vi "convert--duration to formatted string.vi"(1 "duration (seconds)":dbl format="%.3f") -> (0 "duration (formatted string)":string)   [LabVIEW 2020, in "core.lvlib"]
uses:
  core.lvlib
  core_data/chessboard_index.ctl
  core_data/core_data.lvlib
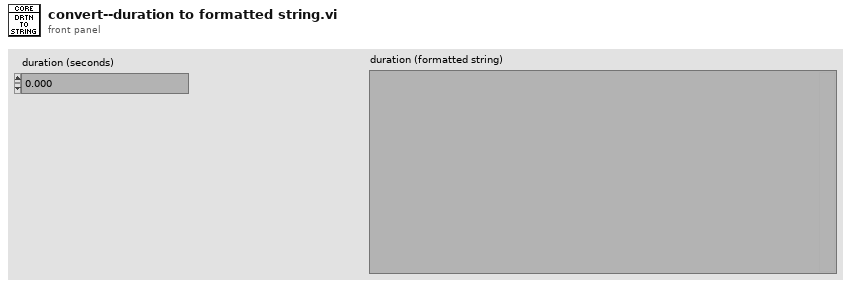
[diagram p1: front panel]
types:
  T1 = typedef "core.lvlib/core_data.lvlib/chessboard_index.ctl" = cluster{"row":u8, "column":u8}
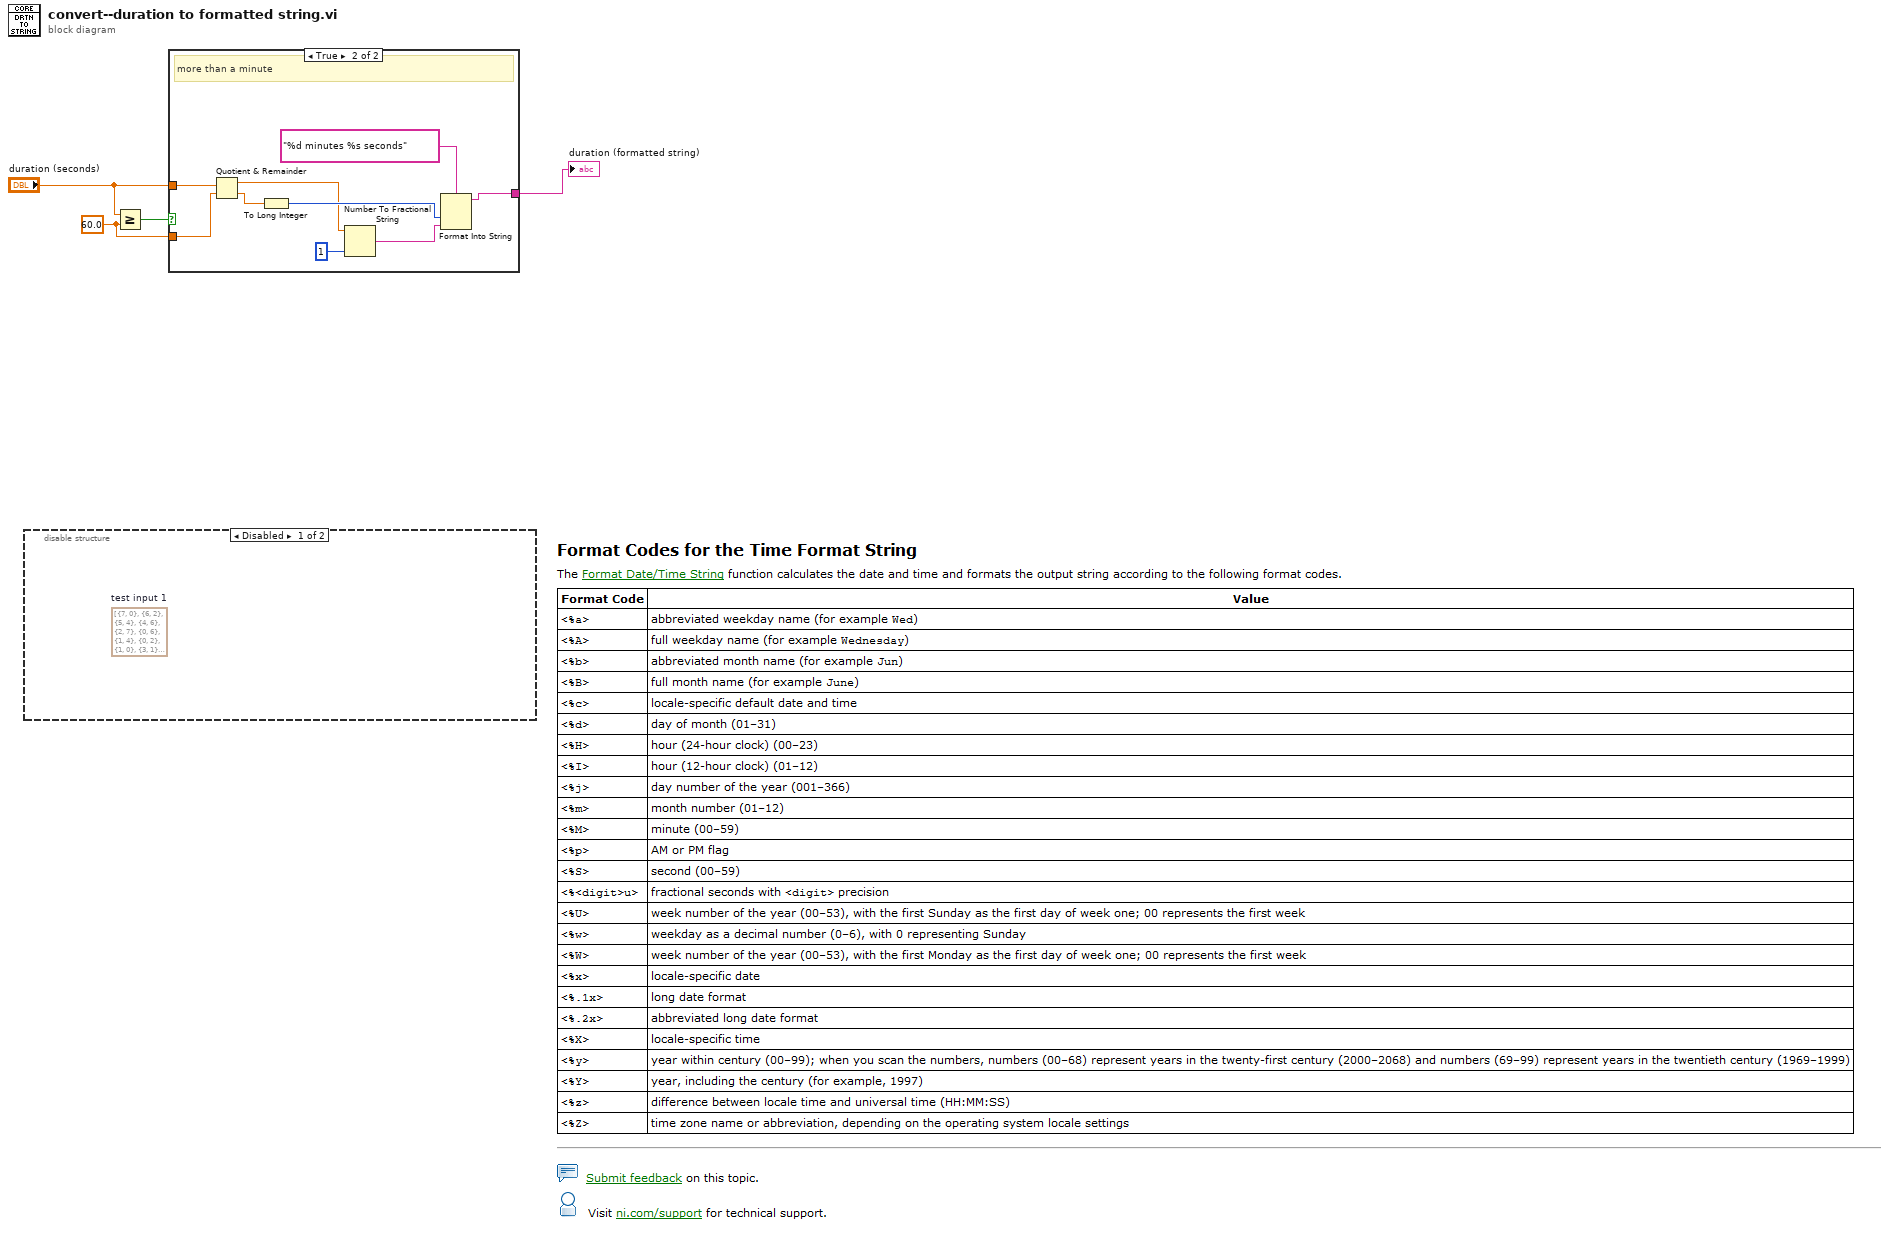
[diagram p0: block diagram]
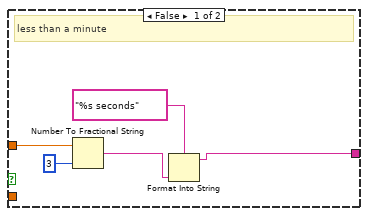
[diagram p2: hidden frame]
diagram:
  w1 = 60.0 ("y")
  n1 = disable-structure shown="Disabled" {
    frame Disabled {
      (unwired) T1[] [{"row"=7, "column"=0}, {"row"=6, "column"=2}, {"row"=5, "column"=4}, {"row"=4, "column"=6}, {"row"=2, "column"=7}, {"row"=0, "column"=6}, {"row"=1, "column"=4}, {"row"=0, "column"=2}, {"row"=1, "column"=0}, {"row"=3, "column"=1}, {"row"=2, "column"=3}, {"row"=1, "column"=5}, {"row"=0, "column"=7}, {"row"=2, "column"=6}, {"row"=0, "column"=5}, {"row"=1, "column"=3}, {"row"=0, "column"=1}, {"row"=2, "column"=0}, {"row"=1, "column"=2}, {"row"=0, "column"=4}, {"row"=2, "column"=5}, {"row"=1, "column"=7}, {"row"=3, "column"=6}, {"row"=2, "column"=4}, {"row"=1, "column"=6}, {"row"=3, "column"=5}, {"row"=4, "column"=3}, {"row"=2, "column"=2}, {"row"=0, "column"=3}, {"row"=1, "column"=1}, {"row"=3, "column"=0}, {"row"=5, "column"=1}, {"row"=3, "column"=2}]  # test input 1
    }
    frame Enabled {
    }
  }
  n2 = Greater Or Equal?(x="duration (seconds)", y=w1) -> (x >= y?=w2:bool)
  n3 = case shown="True" w2 {
    tunnel: "duration (seconds)" -> [w9 w18]
    tunnel: [w5 w10] -> w3
    tunnel: w1 -> [_ w17]
    frame False {
      # "less than a minute"
      n4 = Number To Fractional String(number=w9, precision (6)=i16 3) -> (F-format string=w6:string)  [unwired: 2 in]
      n5 = Format Into String(format string="%s seconds", w6) -> (resulting string=w5:string)  [unwired: 2 in, 1 out]
    }
    frame True {
      # "more than a minute"
      n6 = Quotient & Remainder(x=w18, y=w17) -> (x-y*floor(x/y)=w11:dbl, floor(x/y)=w14:dbl)
      n7 = To Long Integer(number=w14) -> (32bit integer=w12:i32)
      n8 = Number To Fractional String(number=w11, precision (6)=i16 1) -> (F-format string=w13:string)  [unwired: 2 in]
      n9 = Format Into String(format string="%d minutes %s seconds", w12, w13) -> (resulting string=w10:string)  [unwired: 2 in, 1 out]
    }
  }
  "duration (formatted string)" <- w3
